vi "Get LakeShore 340 Set Point.vi"(8 "error in (no error)":errorcluster, 11 "VISA Resource Name":refnum<visa-resource-name>) -> (0 "error out":errorcluster, 2 "Set point":dbl, 3 "VISA Resource Name Out":refnum<visa-resource-name>)   [LabVIEW 2015]
uses:
  GPIB/VISA  Send Receive.vi
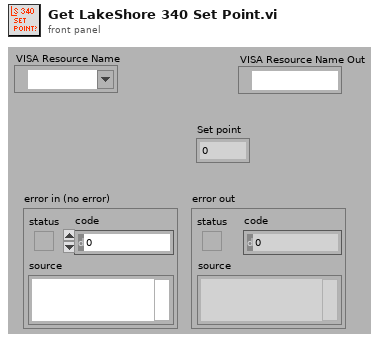
[diagram p1: front panel]
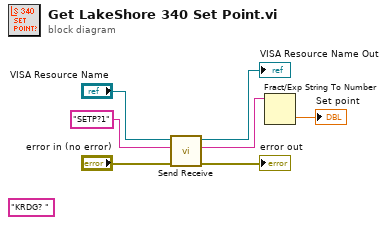
[diagram p0: block diagram]
diagram:
  (unwired) "KRDG? " ("data string in")
  n1 = call-poly "Send Receive.vi"("error in (no error)"="error in (no error)", "data string in"="SETP?1" ("data string"), "VISA Resource Name"="VISA Resource Name") -> ("error out"=→"error out":errorcluster, "data string out"=w6:string, "VISA Resource Name Out"=→"VISA Resource Name Out":refnum<visa-resource-name>)  [unwired: 6 in]
  n2 = Fract/Exp String To Number(string=w6) -> (number=→"Set point":dbl)  [unwired: 4 out]
